vi "DSF.Transceiver.UDP.Set Max Buffer Size.vi"(10 "max buffer size":u64 format="%d bytes", 11 "UDP Transceiver in":refnum<class "DSF.Transceiver.UDP.lvclass">) -> (3 "UDP Transceiver out":refnum<class "DSF.Transceiver.UDP.lvclass">)   [LabVIEW 2017, in "DSF.Transceiver.UDP.lvlib" / "DSF.Transceiver.UDP.lvclass"]
uses:
  DSF.Transceiver.UDP.lvclass
  DSF.Transceiver.UDP.lvclass/DSF.Transceiver.UDP.ctl
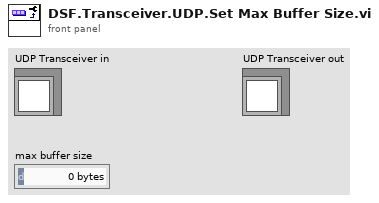
[diagram p1: front panel]
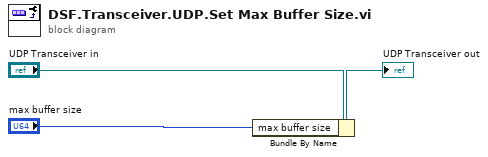
[diagram p0: block diagram]
diagram:
  n1 = Bundle By Name(cluster="UDP Transceiver in", "max buffer size"="max buffer size") -> (→"UDP Transceiver out":refnum<class "DSF.Transceiver.UDP.lvclass">)
